vi "Dequeue Message.vi"(8 "Error In":errorcluster) -> (0 "Error Out":errorcluster, 2 "Data":variant, 3 "State Machine Message":T1)   [LabVIEW 2023, in "QSM - Main.lvlib"]
doc: "This VI dequeues a message from the message queue for the Queued State Machine template."
uses:
  QSM - Main.lvlib
  Controls/State Machine Message.ctl
  Controls/Message Queue Reference Functional Global Variable Operation.ctl
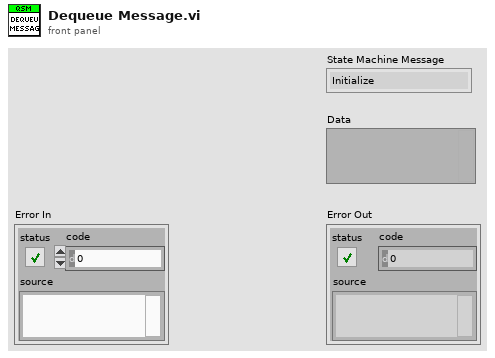
[diagram p1: front panel]
types:
  T1 = typedef "QSM - Main.lvlib/State Machine Message.ctl" = enum16{"Initialize", "Handle Error", "Exit"}
  T2 = typedef "QSM - Main.lvlib/Message Queue Reference Functional Global Variable Operation.ctl" = enum16{"Set", "Get"}
  T3 = typedef "QSM - Library.lvlib/Message Queue Reference.ctl" = refnum<queue>
  T4 = typedef "QSM - Library.lvlib/Message Queue Element.ctl" = cluster{"State Machine Message":T5, "Data":variant}
  T5 = typedef "QSM - Library.lvlib/QSM - State Machine Message.ctl" = enum16{"Initialize", "Handle Error", "Exit"}
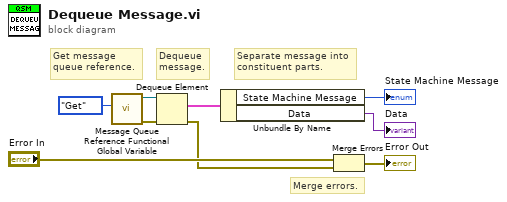
[diagram p0: block diagram]
diagram:
  # "Merge errors."
  # "Separate message into\nconstituent parts."
  # "Dequeue\nmessage."
  # "Get message\nqueue reference."
  n1 = call "Message Queue Reference Functional Global Variable.vi"("Operation"=Message_Queue_Reference_Functional_Global_Variable_Operation."Get") -> ("Error Out"=w9:errorcluster, "Message Queue Reference Out"=w7:T3)  [unwired: 9 in]
  n2 = Dequeue Element(queue=w7, error in (no error)=w9) -> (element=w6:T4, error out=w2:errorcluster)  [unwired: 1 in, 2 out]
  n3 = Unbundle By Name(w6) -> ("State Machine Message"=→"State Machine Message":T5, "Data"=→"Data":variant)
  n4 = Merge Errors("Error In", w2) -> (→"Error Out":errorcluster)
